vi "clear motor error.vi"(8 "error in (no error)":errorcluster, 11 "CL57RS in":refnum<class "CL57RS.lvclass">) -> (0 "error out":errorcluster, 3 "CL57RS out":refnum<class "CL57RS.lvclass">)   [LabVIEW 2025, in "Motor.lvlib" / "CL57RS.lvclass"]
uses:
  CL57RS.lvclass
  CL57RS.lvclass/CL57RS.ctl
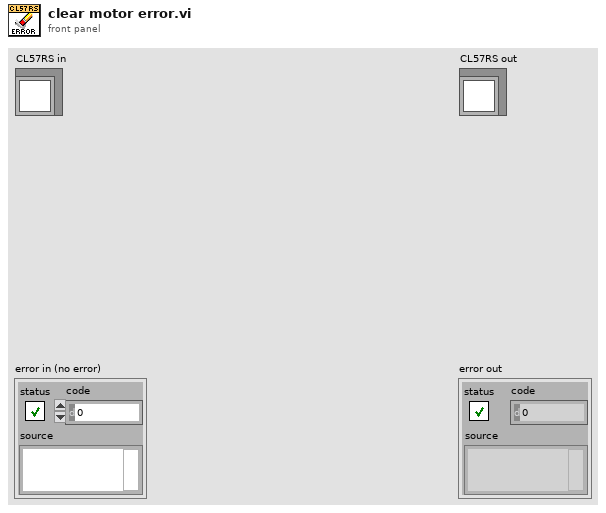
[diagram p1: front panel]
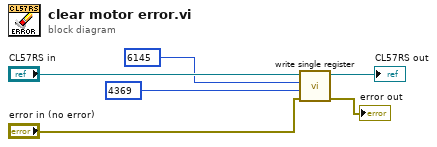
[diagram p0: block diagram]
diagram:
  n1 = call "write single register.vi"("error in (no error)"="error in (no error)", "register to write"=u16 4369, "address"=u16 6145, "CL57RS in"="CL57RS in") -> ("error out"=→"error out":errorcluster, "CL57RS out"=→"CL57RS out":refnum<class "CL57RS.lvclass">)  [unwired: 6 in]
